vi "OPP.AudioStreamer.vi"   [LabVIEW 2020]
uses:
  Typedefs/AudioStreamer.Config.ctl
  Typedefs/AudioStreamer.Config Data.ctl
  Typedefs/AudioStreamer.Signal Data.ctl
  Typedefs/AudioStreamer.Globals.vi
  <vilib>/sound2/lvsound2.llb/Sound Output Write (DBL).vi
types:
  T1 = typedef "AudioStreamer.Config.ctl" = cluster{"Fs (Hz)":dbl, "device":string, "caregiver":cluster{"name":string, "data":dbl[]}, "waver":cluster{"name":string, "data":dbl[]}, "background":cluster{"name":string, "data":dbl[]}, "signal":cluster{"name":string, "data":dbl[]}, "nrep":i32}
  T2 = cluster{enum16{"None", "Start", "Trigger", "Stop"}, "config":T1}
  T3 = typedef "Sound Output Task ID.ctl" = u32
  T4 = typedef "AudioStreamer.Config Data.ctl" = cluster{"device":string, "Fs_Hz":dbl}
  T5 = typedef "AudioStreamer.Signal Data.ctl" = cluster{"destination":string, "name":string, "data":dbl[]}
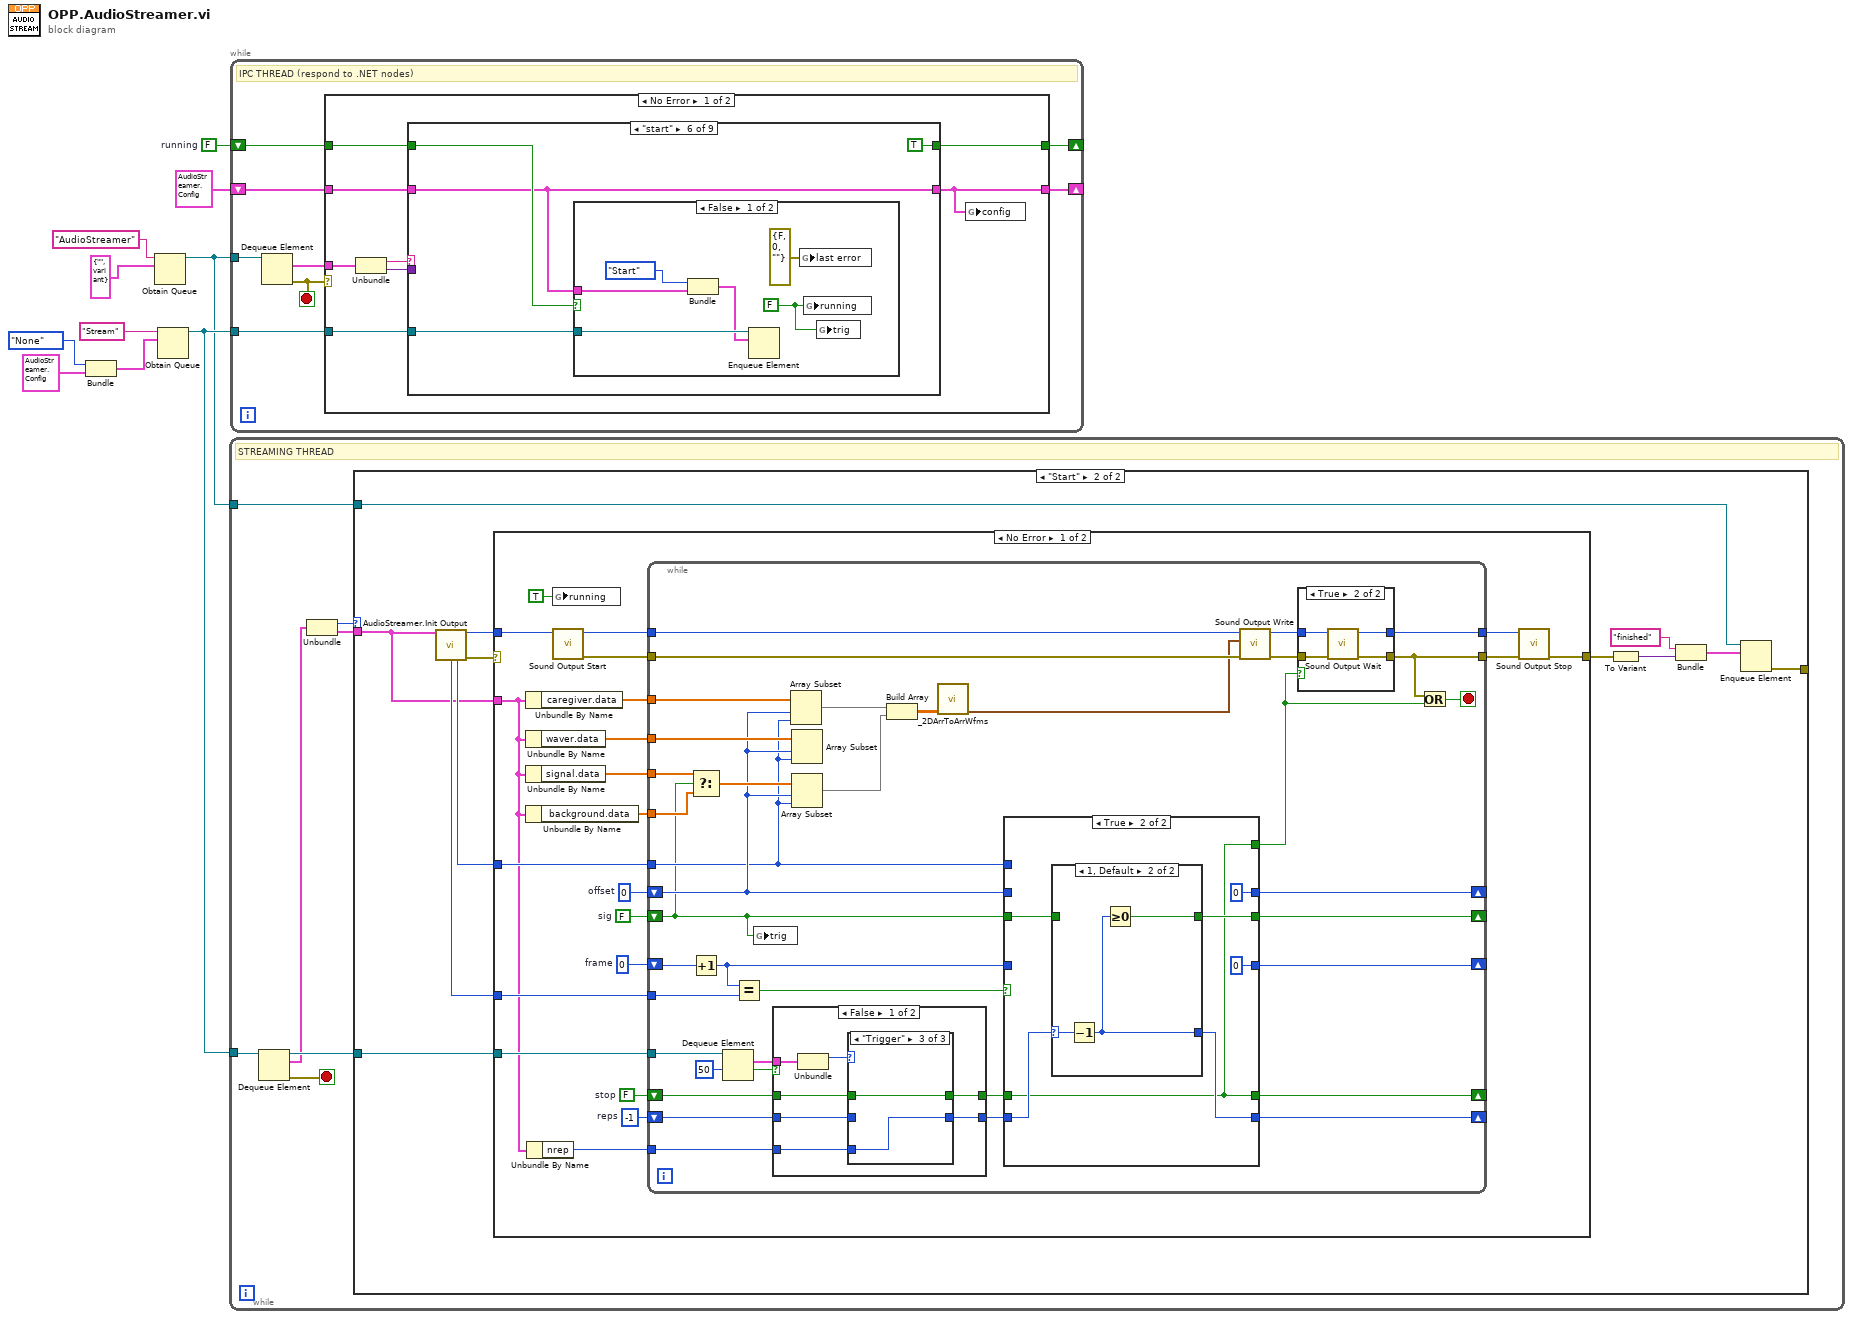
[diagram p0: block diagram]
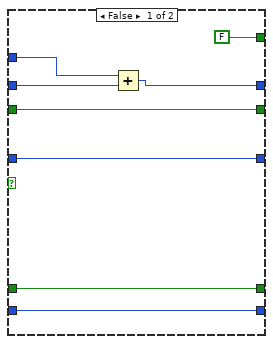
[diagram p3: hidden frame]
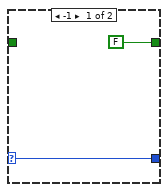
[diagram p4: hidden frame]
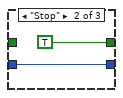
[diagram p7: hidden frame]
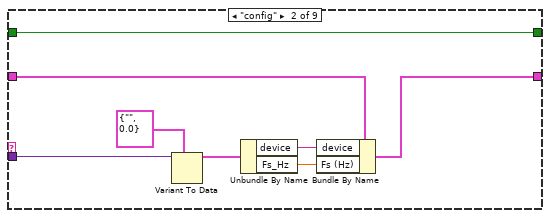
[diagram p11: hidden frame]
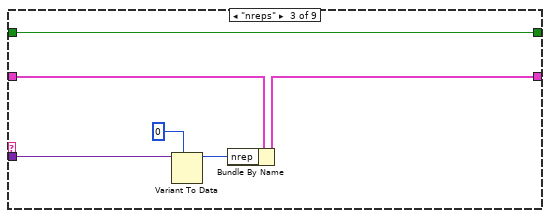
[diagram p12: hidden frame]
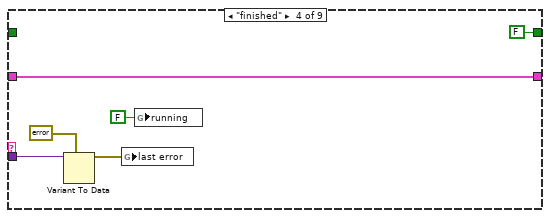
[diagram p13: hidden frame]
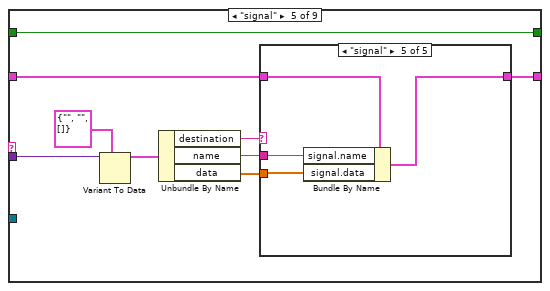
[diagram p14: hidden frame]
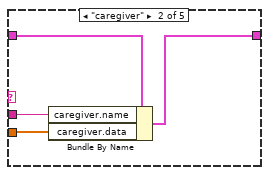
[diagram p16: hidden frame]
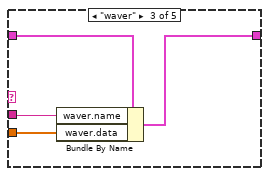
[diagram p17: hidden frame]
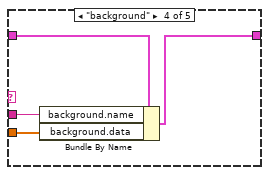
[diagram p18: hidden frame]
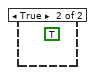
[diagram p19: hidden frame]
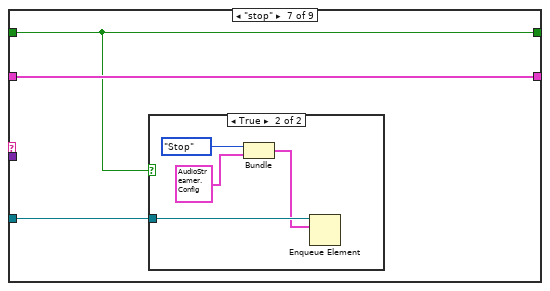
[diagram p20: hidden frame]
diagram:
  w2 = FALSE  # running
  n1 = Bundle(enum16{"None", "Start", "Trigger", "Stop"}."None", "config"=T1 {"Fs (Hz)"=0.0, "device"="", "caregiver"={"name"="", "data"=[]}, "waver"={"name"="", "data"=[]}, "background"={"name"="", "data"=[]}, "signal"={"name"="", "data"=[]}, "nrep"=0}) -> (w3:T2)  [unwired: 1 in]
  n2 = Obtain Queue(name (unnamed)="AudioStreamer", element data type=cluster{string, variant} {"", variant}) -> (queue out=w1:refnum<queue>)  [unwired: 3 in, 2 out]
  n3 = Obtain Queue(name (unnamed)="Stream", element data type=w3) -> (queue out=w7:refnum<queue>)  [unwired: 3 in, 2 out]
  n4 = while {
    tunnel: w7 -> [w17]
    tunnel: w1 -> [w11]
    stop <- w16 stop-if-true
    # "STREAMING THREAD"
    n5 = Dequeue Element(queue=w17) -> (queue out=w15:refnum<queue>, element=w14:T2, error out=w16:errorcluster)  [unwired: 2 in, 1 out]
    n6 = Unbundle(w14) -> (w13:enum16{"None", "Start", "Trigger", "Stop"}, "config"=w12:T1)
    n7 = case shown="\"Start\"" w13 {
      tunnel: w15 -> [_ w28]
      tunnel: w12 -> [_ w18]
      tunnel: w11 -> [_ w25]
      tunnel: [_ w23] -> _
      frame "None", Default {
      }
      frame "Start" {
        n8 = call "AudioStreamer.Init Output.vi"("config"=w18) -> ("task ID"=w22:T3, "framesPerStim"=w19:i32, "ptsPerFrame"=w20:i32, "error out"=w29:errorcluster)  [unwired: 11 in]
        n9 = case shown="No Error" w29 {
          selector: w29 -> [_ w130]
          tunnel: w28 -> [w50 _]
          tunnel: [w43 w130] -> w27
          tunnel: w22 -> [w48 _]
          tunnel: w20 -> [w38 _]
          tunnel: w18 -> [w31 _]
          tunnel: w19 -> [w32 _]
          frame No Error {
            w33 = FALSE  # sig
            w39 = 0  # frame
            w40 = 0  # offset
            w41 = -1  # reps
            w49 = FALSE  # stop
            n10 = Unbundle By Name(w31) -> ("caregiver.data"=w37:dbl[])
            n11 = Unbundle By Name(w31) -> ("waver.data"=w36:dbl[])
            n12 = Unbundle By Name(w31) -> ("signal.data"=w35:dbl[])
            n13 = Unbundle By Name(w31) -> ("background.data"=w34:dbl[])
            n14 = Unbundle By Name(w31) -> ("nrep"=w30:i32)
            n15 = global write "AudioStreamer.Globals.vi" "running"(TRUE ("running")) -> ()
            n16 = call <vilib>:"Sound Output Start.vi"("task ID"=w48) -> ("error out"=w47:errorcluster, "task ID out"=w46:T3)  [unwired: 9 in]
            n17 = while {
              tunnel: w50 -> [w82]
              shift-right: [w55] -> _
              shift-left: w49 -> [w78]
              tunnel: w47 -> [w87]
              tunnel: w46 -> [w88]
              tunnel: [w83] -> w45
              tunnel: [w77] -> w44
              shift-right: [w54] -> _
              shift-left: w41 -> [w75]
              shift-right: [w58] -> _
              shift-left: w40 -> [w62]
              shift-right: [w56] -> _
              shift-left: w39 -> [w73]
              tunnel: w37 -> [w74]
              tunnel: w38 -> [w61]
              tunnel: w36 -> [w72]
              tunnel: w35 -> [w71]
              tunnel: w34 -> [w69]
              shift-right: [w57] -> _
              shift-left: w33 -> [w51]
              tunnel: w32 -> [w65]
              tunnel: w30 -> [w52]
              stop <- w76 stop-if-true
              n18 = Select(t=w71, s=w51, f=w69) -> (s? t:f=w70:dbl[])
              n19 = Increment(x=w73) -> (x+1=w63:i32)
              n20 = Dequeue Element(queue=w82, timeout in ms (-1)=50) -> (element=w79:T2, timed out?=w80:bool)  [unwired: 1 in, 2 out]
              n21 = Equal?(x=w63, y=w65) -> (x = y?=w64:bool)
              n22 = global write "AudioStreamer.Globals.vi" "trig"(w51) -> ()
              n23 = case shown="False" w80 {
                tunnel: w79 -> [w121 _]
                tunnel: w78 -> [w118 w129]
                tunnel: [w119 w129] -> w60
                tunnel: w75 -> [w117 w128]
                tunnel: [w116 w128] -> w59
                tunnel: w52 -> [w115 _]
                frame False {
                  n24 = Unbundle(w121) -> (w120:enum16{"None", "Start", "Trigger", "Stop"})  [unwired: 1 out]
                  n25 = case shown="\"Trigger\"" w120 {
                    tunnel: [w123 TRUE w127] -> w119
                    tunnel: w118 -> [w123 _ w127]
                    tunnel: w117 -> [w122 w124 _]
                    tunnel: [w122 w124 w126] -> w116
                    tunnel: w115 -> [_ _ w126]
                    frame "None", Default {
                    }
                    frame "Stop" {
                    }
                    frame "Trigger" {
                    }
                  }
                }
                frame True {
                }
              }
              n26 = Array Subset(array=w74, index=w62, length=w61) -> (w68:dbl[])
              n27 = Array Subset(array=w72, index=w62, length=w61) -> ()  [unwired: 1 out]
              n28 = Array Subset(array=w70, index=w62, length=w61) -> (w67:dbl[])
              n29 = Build Array(w68, w67) -> (w66:dbl[][])
              n30 = call <vilib>:"_2DArrToArrWfms.vi"("DBL Y"=w66) -> ("data DBL"=w86:waveform(dbl)[])  [unwired: 10 in, 4 out]
              n31 = case shown="True" w64 {
                tunnel: w63 -> [w94 _]
                tunnel: w51 -> [w95 w100]
                tunnel: w62 -> [w96 _]
                tunnel: w61 -> [w90 _]
                tunnel: w60 -> [w93 w97]
                tunnel: w59 -> [w92 w101]
                tunnel: [w91 0 ("offset")] -> w58
                tunnel: [w95 w99] -> w57
                tunnel: [w94 0] -> w56
                tunnel: [w93 w97] -> w55
                tunnel: [w92 w98] -> w54
                tunnel: [FALSE ("stop") w97] -> w53
                frame False {
                  n32 = Add(x=w90, y=w96) -> (x+y=w91:i32)
                }
                frame True {
                  n33 = case shown="1, Default" w101 {
                    selector: w101 -> [w104 w108]
                    tunnel: w100 -> [_ _]
                    tunnel: [FALSE w106] -> w99
                    tunnel: [w104 w107] -> w98
                    frame -1 {
                    }
                    frame 1, Default {
                      n34 = Decrement(x=w108) -> (x-1=w107:i32)
                      n35 = Greater Or Equal To 0?(x=w107) -> (x >= 0?=w106:bool)
                    }
                  }
                }
              }
              n36 = call-poly <vilib>:"Sound Output Write.vi"("error in (no error)"=w87, "data"=w86, "task ID"=w88) -> ("error out"=w85:errorcluster, "task ID out"=w84:T3)  [unwired: 7 in]
              n37 = case shown="True" w53 {
                tunnel: w85 -> [w109 w114]
                tunnel: w84 -> [w110 w113]
                tunnel: [w110 w112] -> w83
                tunnel: [w109 w111] -> w77
                frame False {
                }
                frame True {
                  n38 = call <vilib>:"Sound Output Wait.vi"("error in (no error)"=w114, "task ID"=w113) -> ("error out"=w111:errorcluster, "task ID out"=w112:T3)  [unwired: 8 in]
                }
              }
              n39 = Or(x=w77, y=w53) -> (x .or. y?=w76:bool)
            }
            n40 = call <vilib>:"Sound Output Stop.vi"("error in (no error)"=w44, "task ID"=w45) -> ("error out"=w43:errorcluster)  [unwired: 8 in, 1 out]
          }
          frame Error {
          }
        }
        n41 = To Variant(anything=w27) -> (Variant=w21:variant)
        n42 = Bundle("finished", "Variant"=w21) -> (w24:cluster{string, "Variant":variant})  [unwired: 1 in]
        n43 = Enqueue Element(queue=w25, element=w24) -> (error out=w23:errorcluster)  [unwired: 2 in, 2 out]
      }
    }
  }
  n44 = while {
    tunnel: w1 -> [w138]
    tunnel: w7 -> [w135]
    shift-right: [w133] -> _
    shift-left: T1 {"Fs (Hz)"=0.0, "device"="", "caregiver"={"name"="", "data"=[]}, "waver"={"name"="", "data"=[]}, "background"={"name"="", "data"=[]}, "signal"={"name"="", "data"=[]}, "nrep"=0} ("config") -> [w134]
    shift-right: [w131] -> _
    shift-left: w2 -> [w132]
    stop <- w137 stop-if-true
    # "IPC THREAD (respond to .NET nodes)"
    n45 = Dequeue Element(queue=w138) -> (element=w136:cluster{string, variant}, error out=w137:errorcluster)  [unwired: 2 in, 2 out]
    n46 = case shown="No Error" w137 {
      tunnel: w136 -> [w146 _]
      tunnel: w135 -> [w143 _]
      tunnel: w134 -> [w142 w222]
      tunnel: [w139 w222] -> w133
      tunnel: w132 -> [w141 w221]
      tunnel: [w140 w221] -> w131
      frame No Error {
        n47 = Unbundle(w146) -> (w145:string, w144:variant)
        n48 = case shown="\"start\"" w145 {
          tunnel: w144 -> [_ w156 w162 w167 w177 _ _ _ _]
          tunnel: w143 -> [_ _ _ _ _ w198 w206 w213 _]
          tunnel: w142 -> [w148 w153 w161 w168 w174 w195 w207 w214 w220]
          tunnel: [w148 w150 w160 w168 w173 w195 w207 w214 w220] -> w139
          tunnel: w141 -> [w147 w149 w159 _ w170 w197 w205 w212 w219]
          tunnel: [w147 w149 w159 FALSE ("running") w170 TRUE w205 w212 w219] -> w140
          frame "", Default {
          }
          frame "config" {
            n49 = Variant To Data(type=T4 {"device"="", "Fs_Hz"=0.0} ("config data"), Variant=w156) -> (data=w154:T4)  [unwired: 1 in, 1 out]
            n50 = Unbundle By Name(w154) -> ("device"=w152:string, "Fs_Hz"=w151:dbl)
            n51 = Bundle By Name(cluster=w153, "device"=w152, "Fs (Hz)"=w151) -> (w150:T1)
          }
          frame "nreps" {
            n52 = Variant To Data(type=0, Variant=w162) -> (data=w157:i32)  [unwired: 1 in, 1 out]
            n53 = Bundle By Name(cluster=w161, "nrep"=w157) -> (w160:T1)
          }
          frame "finished" {
            n54 = Variant To Data(type=errorcluster {"status"=FALSE, "code"=0, "source"=""} ("error constant"), Variant=w167) -> (data=w163:errorcluster)  [unwired: 1 in, 1 out]
            n55 = global write "AudioStreamer.Globals.vi" "last error"(w163) -> ()
            n56 = global write "AudioStreamer.Globals.vi" "running"(FALSE ("running")) -> ()
          }
          frame "signal" {
            n57 = Variant To Data(type=T5 {"destination"="", "name"="", "data"=[]} ("signal data"), Variant=w177) -> (data=w175:T5)  [unwired: 1 in, 1 out]
            n58 = Unbundle By Name(w175) -> ("destination"=w172:string, "name"=w171:string, "data"=w169:dbl[])
            n59 = case shown="\"signal\"" w172 {
              tunnel: w174 -> [w178 w182 w186 w190 w194]
              tunnel: [w178 w181 w185 w189 w193] -> w173
              tunnel: w171 -> [_ w180 w184 w188 w192]
              tunnel: w169 -> [_ w179 w183 w187 w191]
              frame "", Default {
              }
              frame "caregiver" {
                n60 = Bundle By Name(cluster=w182, "caregiver.name"=w180, "caregiver.data"=w179) -> (w181:T1)
              }
              frame "waver" {
                n61 = Bundle By Name(cluster=w186, "waver.name"=w184, "waver.data"=w183) -> (w185:T1)
              }
              frame "background" {
                n62 = Bundle By Name(cluster=w190, "background.name"=w188, "background.data"=w187) -> (w189:T1)
              }
              frame "signal" {
                n63 = Bundle By Name(cluster=w194, "signal.name"=w192, "signal.data"=w191) -> (w193:T1)
              }
            }
          }
          frame "start" {
            n64 = case shown="False" w197 {
              tunnel: w195 -> [w204 _]
              tunnel: w198 -> [w202 _]
              frame False {
                w199 = FALSE ("running")
                n65 = Bundle(enum16{"None", "Start", "Trigger", "Stop"}."Start", "config"=w204) -> (w201:T2)  [unwired: 1 in]
                n66 = Enqueue Element(queue=w202, element=w201) -> ()  [unwired: 2 in, 3 out]
                n67 = global write "AudioStreamer.Globals.vi" "last error"(errorcluster {"status"=FALSE, "code"=0, "source"=""} ("last error")) -> ()
                n68 = global write "AudioStreamer.Globals.vi" "running"(w199) -> ()
                n69 = global write "AudioStreamer.Globals.vi" "trig"(w199) -> ()
              }
              frame True {
                (unwired) TRUE
              }
            }
          }
          frame "stop" {
            n70 = case shown="True" w205 {
              tunnel: w206 -> [_ w210]
              frame False {
              }
              frame True {
                n71 = Bundle(enum16{"None", "Start", "Trigger", "Stop"}."Stop", "config"=T1 {"Fs (Hz)"=0.0, "device"="", "caregiver"={"name"="", "data"=[]}, "waver"={"name"="", "data"=[]}, "background"={"name"="", "data"=[]}, "signal"={"name"="", "data"=[]}, "nrep"=0}) -> (w209:T2)  [unwired: 1 in]
                n72 = Enqueue Element(queue=w210, element=w209) -> ()  [unwired: 2 in, 3 out]
              }
            }
          }
          frame "trigger" {
            n73 = case shown="True" w212 {
              tunnel: w213 -> [_ w217]
              frame False {
              }
              frame True {
                n74 = Bundle(enum16{"None", "Start", "Trigger", "Stop"}."Trigger", "config"=T1 {"Fs (Hz)"=0.0, "device"="", "caregiver"={"name"="", "data"=[]}, "waver"={"name"="", "data"=[]}, "background"={"name"="", "data"=[]}, "signal"={"name"="", "data"=[]}, "nrep"=0}) -> (w216:T2)  [unwired: 1 in]
                n75 = Enqueue Element(queue=w217, element=w216) -> ()  [unwired: 2 in, 3 out]
              }
            }
          }
          frame "close" {
          }
        }
        n76 = global write "AudioStreamer.Globals.vi" "config"(w139) -> ()
      }
      frame Error {
      }
    }
  }
